vi "G#Object_ConvertFlattenedDataToMoreGeneric.vi"(0 "reference in":refnum<class "G#Object.lvclass">, 1 "full class name":string, 3 "type string":i16[](array[numeric]), 5 "error in (no error)":errorcluster) -> (14 "reference converterrd":refnum<class "G#Object.lvclass">, 19 "error out":errorcluster)   [LabVIEW 2017, in "G#Object.lvclass"]
doc: "Converts the reference in to the more generic class specifiec by the full class name."
uses:
  G#Object.lvclass
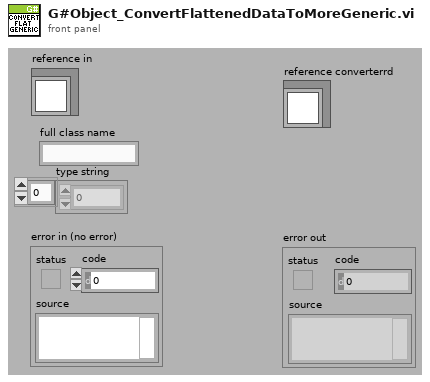
[diagram p1: front panel]
types:
  T1 = typedef "G#Object.lvclass/G#Object_ClassHierarchy.ctl" = cluster{"ClassName":string, "FullClassName":string, "ClassPath":path, "IsLeaf":bool}
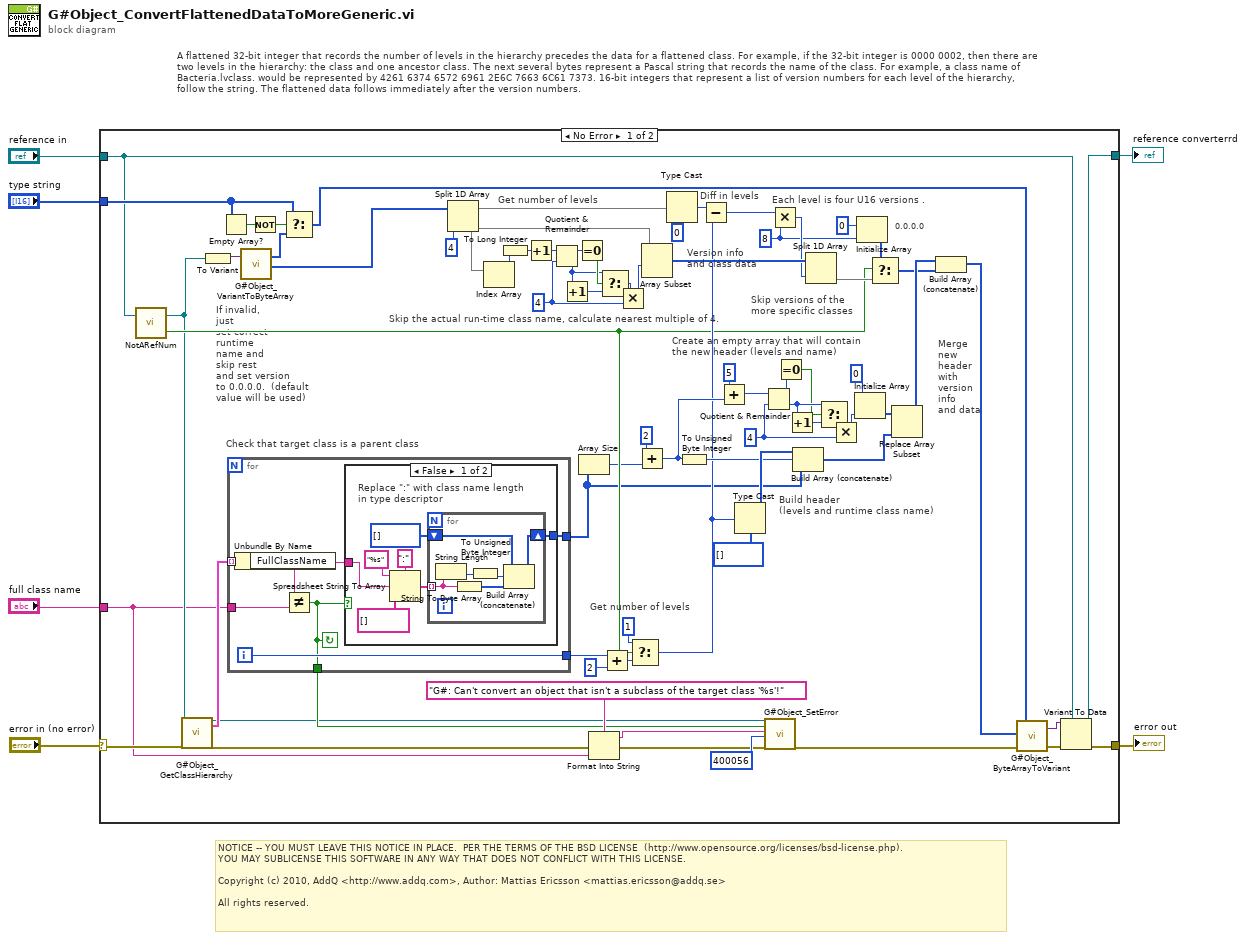
[diagram p0: block diagram]
diagram:
  # "A flattened 32-bit integer that records the number of levels in the hierarchy precedes the data for a flattened class. For example, if the 32-bit integer is 0000 0002, then there are two levels in the hierarchy: the class and one ancestor class. The next several bytes represent a Pascal string that records the name of the class. For example, a class name of Bacteria.lvclass. would be represented by 4261 6374 6572 6961 2E6C 7663 6C61 7373. 16-bit integers that represent a list of version numbers for each level of the hierarchy, follow the string. The flattened data follows immediately after the version numbers."
  # "NOTICE -- YOU MUST LEAVE THIS NOTICE IN PLACE.  PER THE TERMS OF THE BSD LICENSE  (http://www.opensource.org/licenses/bsd-license.php).\nYOU MAY SUBLICENSE THIS SOFTWARE IN ANY WAY THAT DOES NOT CONFLICT WITH THIS LICENSE.\n\nCopyright (c) 2010, AddQ <http://www.addq.com>, Author: Mattias Ericsson <mattias.ericsson@addq.se>\n\nAll rights reserved."
  n1 = case shown="No Error" "error in (no error)" {
    selector: "error in (no error)" -> [w30 w101]
    tunnel: [w26 w101] -> w4
    tunnel: "full class name" -> [w15 _]
    tunnel: "reference in" -> [w25 w100]
    tunnel: "type string" -> [w27 _]
    tunnel: [w24 w100] -> w1
    frame No Error {
      w47 = 4 ("y")
      w35 = 8 ("y")
      w50 = 4 ("y")
      # "0.0.0.0"
      # "If invalid,\njust\nset correct\nruntime\nname and\nskip rest\nand set version\nto 0.0.0.0.  (default\nvalue will be used)"
      # "Each level is four U16 versions ."
      # "Merge\nnew\nheader\nwith\nversion\ninfo\nand data"
      # "Build header\n(levels and runtime class name)"
      # "Create an empty array that will contain\nthe new header (levels and name)"
      # "Skip versions of the\nmore specific classes"
      # "Diff in levels"
      # "Get number of levels"
      # "Version info\nand class data"
      # "Skip the actual run-time class name, calculate nearest multiple of 4."
      # "Get number of levels"
      # "Check that target class is a parent class"
      n2 = call-dynamic "NotARefNum.vi"("reference in"=w25) -> ("not a refnum?"=w36:bool, "reference out"=w17:refnum<class "G#Object.lvclass">)  [unwired: 1 in]
      n3 = call "G#Object_GetClassHierarchy.vi"("reference in"=w17, "error in (no error)"=w30) -> ("reference out"=w16:refnum<class "G#Object.lvclass">, "class hierarchy"=w80:T1[], "error out"=w19:errorcluster)  [unwired: 15 in]
      n4 = To Variant(anything=w17) -> (Variant=w14:variant)
      n5 = Empty Array?(array=w27) -> (empty?=w29:bool)
      n6 = for {
        tunnel: w80 -> [w86] mode=indexing
        tunnel: w15 -> [w83]
        tunnel: [w85] -> w79
        tunnel: [w84] -> w18
        tunnel: [w81] -> w32
        i -> [w85]
        stop <- w84 continue-if-true
        n7 = Unbundle By Name(w86) -> ("FullClassName"=w82:string)
        n8 = Not Equal?(x=w82, y=w83) -> (x != y?=w84:bool)
        n9 = case shown="False" w84 {
          tunnel: w82 -> [w91 _]
          tunnel: [w87 _] -> w81
          frame False {
            # "Replace \":\" with class name length\nin type descriptor"
            n10 = Spreadsheet String To Array(delimiter (Tab)=":", format string="%s", spreadsheet string=w91, array type (2D Dbl)=string[] []) -> (array=w89:string[])
            n11 = for {
              tunnel: w89 -> [w98] mode=indexing
              shift-right: [w95] -> w87
              shift-left: u8[] [] -> [w94]
              n12 = String Length(string=w98) -> (length=w99:i32)
              n13 = String To Byte Array(string=w98) -> (unsigned byte array=w96:u8[])
              n14 = To Unsigned Byte Integer(number=w99) -> (unsigned 8bit integer=w97:u8)
              n15 = Build Array (concatenate)(w94, w97, w96) -> (w95:u8[])
            }
          }
          frame True {
          }
        }
      }
      n16 = call "G#Object_VariantToByteArray.vi"("variant"=w14) -> ("type string"=w13:i16[], "unsigned byte array"=w12:u8[])  [unwired: 17 in]
      n17 = Not(x=w29) -> (.not. x?=w28:bool)
      n18 = Select(t=w27, s=w28, f=w13) -> (s? t:f=w11:i16[])
      n19 = Split 1D Array(array=w12, index=4 ("length")) -> (first subarray=w70:u8[], second subarray=w44:u8[])
      n20 = Index Array(array=w44) -> (element=w77:u8)  [unwired: 1 in]
      n21 = To Long Integer(number=w77) -> (32bit integer=w43:i32)
      n22 = Increment(x=w43) -> (x+1=w42:i32)
      n23 = Quotient & Remainder(x=w42, y=w50) -> (x-y*floor(x/y)=w76:i32, floor(x/y)=w73:i32)
      n24 = Increment(x=w73) -> (x+1=w74:i32)
      n25 = Equal To 0?(x=w76) -> (x = 0?=w75:bool)
      n26 = Array Size(array=w32) -> (size(s)=w31:i32)
      n27 = Format Into String(format string="G#: Can't convert an object that isn't a subclass of the target class '%s'!", error in=w19, w15) -> (resulting string=w20:string, error out=w21:errorcluster)  [unwired: 1 in]
      n28 = Select(t=w73, s=w75, f=w74) -> (s? t:f=w52:i32)
      n29 = Add(x=w79, y=2) -> (x+y=w41:i32)
      n30 = Multiply(x=w52, y=w50) -> (x*y=w51:i32)
      n31 = Select(t=1, s=w36, f=w41) -> (s? t:f=w40:i32)
      n32 = Add(x=2, y=w31) -> (x+y=w58:i32)
      n33 = Array Subset(array=w44, index=w51) -> (w66:u8[])  [unwired: 1 in]
      n34 = Type Cast(type=0 ("y"), x=w70) -> (*(type *) &x=w68:i32)
      n35 = To Unsigned Byte Integer(number=w58) -> (unsigned 8bit integer=w57:u8)
      n36 = Subtract(x=w68, y=w40) -> (x-y=w67:i32)
      n37 = Add(x=5, y=w58) -> (x+y=w60:i32)
      n38 = Type Cast(type=u8[] [] ("unsigned byte array"), x=w40) -> (*(type *) &x=w59:u8[])
      n39 = Quotient & Remainder(x=w60, y=w47) -> (x-y*floor(x/y)=w61:i32, floor(x/y)=w64:i32)
      n40 = call "G#Object_SetError.vi"("reference in"=w16, "error (F)"=w18, "source"=w20, "code"=400056, "error in (no error)"=w21) -> ("error out"=w8:errorcluster)  [unwired: 14 in]
      n41 = Multiply(x=w67, y=w35) -> (x*y=w46:i32)
      n42 = Equal To 0?(x=w61) -> (x = 0?=w62:bool)
      n43 = Increment(x=w64) -> (x+1=w63:i32)
      n44 = Build Array (concatenate)(w59, w57, w32) -> (w54:u8[])
      n45 = Split 1D Array(array=w66, index=w46) -> (second subarray=w38:u8[])  [unwired: 1 out]
      n46 = Select(t=w64, s=w62, f=w63) -> (s? t:f=w49:i32)
      n47 = Multiply(x=w49, y=w47) -> (x*y=w48:i32)
      n48 = Initialize Array(u8 0, w48) -> (w55:u8[])
      n49 = Initialize Array(u8 0, w35) -> (w34:u8[])
      n50 = Select(t=w34, s=w36, f=w38) -> (s? t:f=w37:u8[])
      n51 = Replace Array Subset(array=w55, new element=w54) -> (w53:u8[])  [unwired: 1 in]
      n52 = Build Array (concatenate)(w53, w37) -> (w10:u8[])
      n53 = call "G#Object_ByteArrayToVariant.vi"("unsigned byte array"=w10, "error in"=w8, "type string"=w11) -> ("variant"=w9:variant, "error out"=w7:errorcluster)  [unwired: 15 in]
      n54 = Variant To Data(error in=w7, type=w25, Variant=w9) -> (data=w24:refnum<class "G#Object.lvclass">, error out=w26:errorcluster)
    }
    frame Error {
    }
  }
  "error out" <- w4
  "reference converterrd" <- w1
